vi "T触发器(JK下降沿-T).vi"(1 "CP":bool, 2 "T":bool) -> (0 "Q":bool)   [LabVIEW 2012, in "触发器.lvlib"]
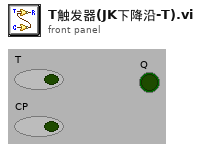
[diagram p1: front panel]
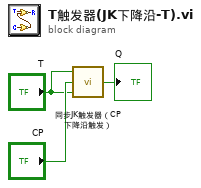
[diagram p0: block diagram]
diagram:
  n1 = call "同步JK触发器（CP下降沿触发）.vi"("k"="T", "c"="CP", "J"="T") -> ("Q"=→"Q":bool)
